vi "gfitsio-read-column-variant.vi"(7 "column":string, 8 "error in (no error)":errorcluster, 9 "row":i32, 11 "gfits refnum":T1) -> (0 "error out":errorcluster, 2 "data":variant, 3 "dup gfits refnum":T1)   [LabVIEW 2019, in "gfitsio.lvlib"]
doc: "Read elements from an ASCII or binary table column."
uses:
  gfitsio.lvlib
  gfitsio-refnum.ctl
  cfitsio-datatypes.ctl
  <vilib>/Utility/VariantDataType/MemoryInfo.ctl
  <vilib>/Utility/VariantDataType/MemoryType.ctl
  <vilib>/Utility/VariantDataType/VariantType.lvlib
  gfitsio.dll
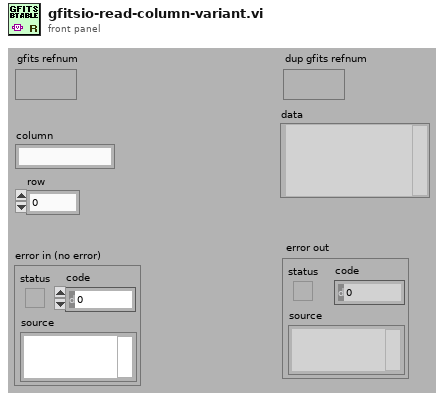
[diagram p1: front panel]
types:
  T1 = typedef "gfitsio.lvlib/gfitsio-refnum.ctl" = refnum<k1>
  T2 = typedef "gfitsio.lvlib/cfitsio-datatypes.ctl" = i32
  T3 = enum16{"big-endian, network order", "native, host order", "little-endian"}
  T4 = typedef "VariantType.lvlib/MemoryInfo.ctl" = cluster{"Type":T5, "Size":u32}
  T5 = typedef "VariantType.lvlib/MemoryType.ctl" = enum16{"Variable", "Fixed", "Bounded"}
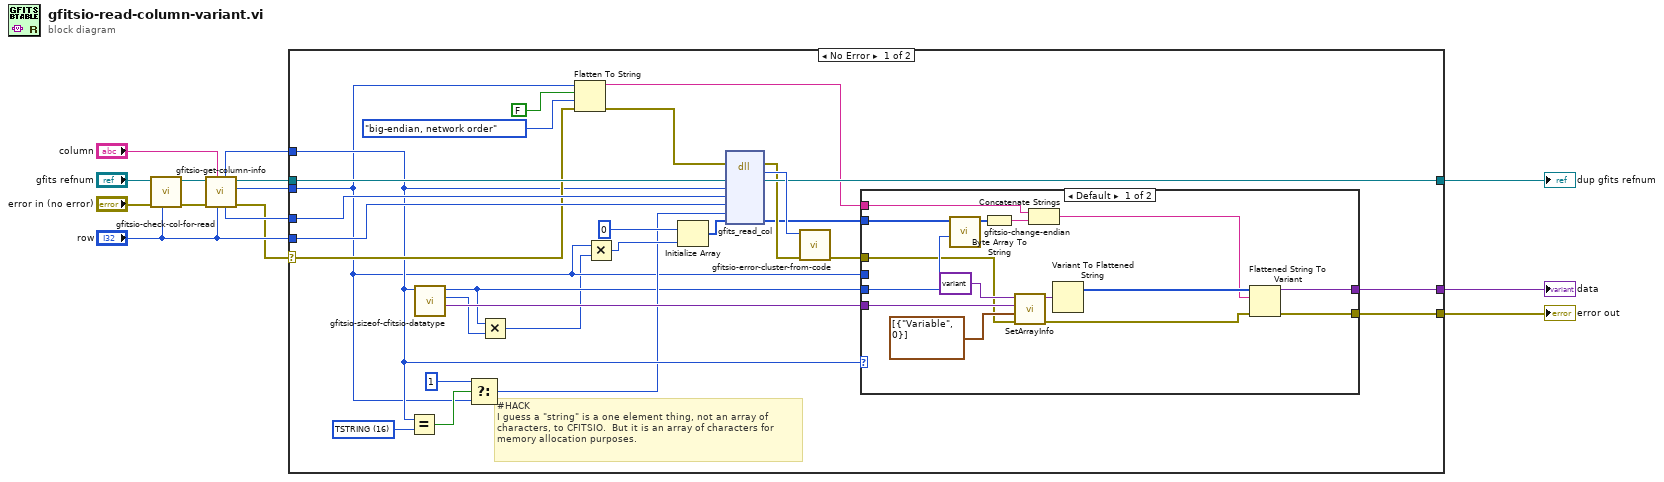
[diagram p0: block diagram]
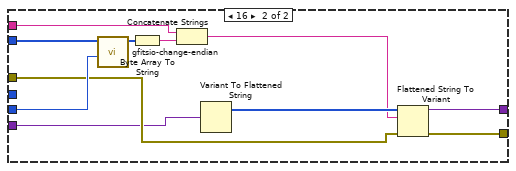
[diagram p2: hidden frame]
diagram:
  n1 = call "gfitsio-check-col-for-read.vi"("row"="row", "error in (no error)"="error in (no error)", "gfits refnum"="gfits refnum") -> ("error out"=w4:errorcluster, "dup gfits refnum"=w3:T1)  [unwired: 4 in, 3 out]
  n2 = call "gfitsio-get-column-info.vi"("row (-1: don't check descriptor)"="row", "column"="column", "error in (no error)"=w4, "gfits refnum"=w3) -> ("error out"=w2:errorcluster, "nelements"=w7:i32, "dup gfits refnum"=w1:T1, "column number"=w8:i32, "cfitsio datatype"=w9:T2)  [unwired: 2 in, 1 out]
  n3 = case shown="No Error" w2 {
    selector: w2 -> [w29 w70]
    tunnel: [w26 w70] -> w13
    tunnel: w1 -> [w40 w69]
    tunnel: [w41 w69] -> w12
    tunnel: "row" -> [w39 _]
    tunnel: [w30 _] -> w14
    tunnel: w7 -> [w19 _]
    tunnel: w8 -> [w37 _]
    tunnel: w9 -> [w22 _]
    frame No Error {
      w23 = T2 16 items=["TBIT"=1, "TBYTE  (U8)"=11, "TSBYTE  (I8)"=12, "TLOGICAL"=14, "TSTRING"=16, "TUSHORT  (U16)"=20, "TSHORT  (I16)"=21, "TUINT"=31, "TULONG  (U32)"=40, "TLONG  (I32)"=41, "TFLOAT  (SGL)"=42, "TLONGLONG  (I64)"=81, "TDOUBLE  (DBL)"=82, "TCOMPLEX  (CSG)"=83, "TDOUBLECOMPLEX  (CDB)"=163] ("cfitsio datatype")
      # "#HACK\nI guess a \"string\" is a one element thing, not an array of characters, to CFITSIO.  But it is an array of characters for memory allocation purposes."
      n4 = Equal?(x=w22, y=w23) -> (x = y?=w21:bool)
      n5 = call "gfitsio-sizeof-cfitsio-datatype.vi"("cfitsio datatype"=w22) -> ("Variant datatype"=w35:variant, "words/element"=w16:i32, "size (bytes)"=w17:i32)  [unwired: 8 in]
      n6 = Select(t=1, s=w21, f=w19) -> (s? t:f=w20:i32)
      n7 = Multiply(x=w17, y=w16) -> (x*y=w15:i32)
      n8 = Flatten To String(anything=w19, prepend array or string size? (T)=FALSE ("data includes array or string size? (T)"), byte order (0:big-endian, network order)=T3."big-endian, network order", error in (no error)=w29) -> (data string=w32:string, error out=w28:errorcluster)  [unwired: 1 out]
      n9 = Multiply(x=w19, y=w15) -> (x*y=w25:i32)
      n10 = Initialize Array(u8 0 ("element"), w25) -> (w24:u8[])
      n11 = dll-call lib="C:/Users/ggatling/local/GFITSIO/gfitsio/gfitsio.dll" fn="gfits_read_col"(error in=w28, "refnum"=w40, "datatype"=w22, "colnum"=w37, "row"=w39, "nelements"=w20, "data"=w24) -> (error out=w36:errorcluster, "return type"=w42:i32, "refnum"=w41:T1, "data"=w31:u8[])  [unwired: 6 in, 1 out]
      n12 = call "gfitsio-error-cluster-from-code.vi"("error in (no error)"=w36, "error code"=w42) -> ("error out"=w27:errorcluster)  [unwired: 9 out]
      n13 = case shown="Default" w22 {
        tunnel: w17 -> [w56 w67]
        tunnel: w35 -> [w53 w58]
        tunnel: w19 -> [_ _]
        tunnel: w32 -> [w49 w64]
        tunnel: w31 -> [w48 w63]
        tunnel: [w47 w62] -> w30
        tunnel: w27 -> [w45 w59]
        tunnel: [w44 w61] -> w26
        frame Default {
          n14 = call "gfitsio-change-endian.vi"("word size (bytes)"=w56, "data in"=w48) -> ("data out"=w57:u8[])  [unwired: 9 in]
          n15 = Byte Array To String(unsigned byte array=w57) -> (string=w50:string)
          n16 = call <vilib>:"SetArrayInfo.vi"("error in (no error)"=w45, "Array Lengths"=T4[] [{"Type"=enum."Variable", "Size"=0}], "Array Element"=w53, "Variant"=variant(u8[] []) ("variant 2")) -> ("error out"=w46:errorcluster, "Variant Out"=w51:variant)  [unwired: 6 in]
          n17 = Concatenate Strings(w49, w50) -> (w43:string)
          n18 = Variant To Flattened String(Variant=w51) -> (1:w52:i16[])  [unwired: 1 out]
          n19 = Flattened String To Variant(4:w46, 6:w43, 7:w52) -> (0:w44:errorcluster, 3:w47:variant)
        }
        frame 16 {
          n20 = call "gfitsio-change-endian.vi"("word size (bytes)"=w67, "data in"=w63) -> ("data out"=w68:u8[])  [unwired: 9 in]
          n21 = Byte Array To String(unsigned byte array=w68) -> (string=w65:string)
          n22 = Concatenate Strings(w64, w65) -> (w60:string)
          n23 = Variant To Flattened String(Variant=w58) -> (1:w66:i16[])  [unwired: 1 out]
          n24 = Flattened String To Variant(4:w59, 6:w60, 7:w66) -> (0:w61:errorcluster, 3:w62:variant)
        }
      }
    }
    frame Error {
    }
  }
  "error out" <- w13
  "dup gfits refnum" <- w12
  "data" <- w14
